vi "SetGreenLevel.vi"(8 "error in":errorcluster, 10 "Numeric":sgl) -> (0 "error out":errorcluster)   [LabVIEW 2010]
uses:
  <userlib>/ROSforLV_0.1/ROS/MessageBuilding/Primitives/subs/float32Scalar.vi
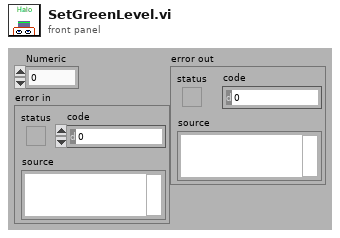
[diagram p1: front panel]
types:
  T1 = typedef "_ROSControl.ctl" = cluster{"topic port":u16, "Node":string, "topic":string, "type":string, "node port":u32, "error ":errorcluster, "Direction":T2, "APIs":string[]}
  T2 = typedef "_ROSDirection.ctl" = enum16{"Node", "Publisher", "Subscriber", "Service Client"}
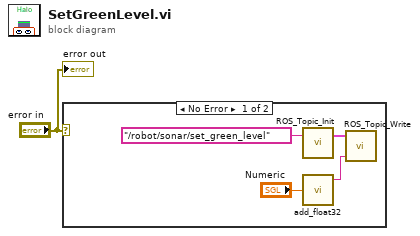
[diagram p0: block diagram]
diagram:
  n1 = case shown="No Error" "error in" {
    frame No Error {
      n2 = call <userlib>:"ROS_Topic_Init.vi"("topic"="/robot/sonar/set_green_level") -> ("ROS out"=w5:T1)  [unwired: 2 in]
      n3 = call-poly <userlib>:"add_float32.vi"("Numeric"="Numeric") -> ("msg out"=w3:string)  [unwired: 4 in]
      n4 = call <userlib>:"ROS_Topic_Write.vi"("Msg in"=w3, "ROS in"=w5) -> ()  [unwired: 2 in, 1 out]
    }
    frame Error {
    }
  }
  "error out" <- "error in"
